vi "Plot_RT_Graph.vi"() -> ()   [LabVIEW 2017]
uses:
  <vilib>/Utility/file.llb/Read From Spreadsheet File (DBL).vi
panel:
  out "R vs T":cluster{"all rows":dbl[], "all rows":dbl[]}(graph)
  in  "stop":bool
  out "T vs t":cluster{"all rows":dbl[], "all rows":dbl[]}(graph)
  in  "file path X":path=path "c:/test.txt"
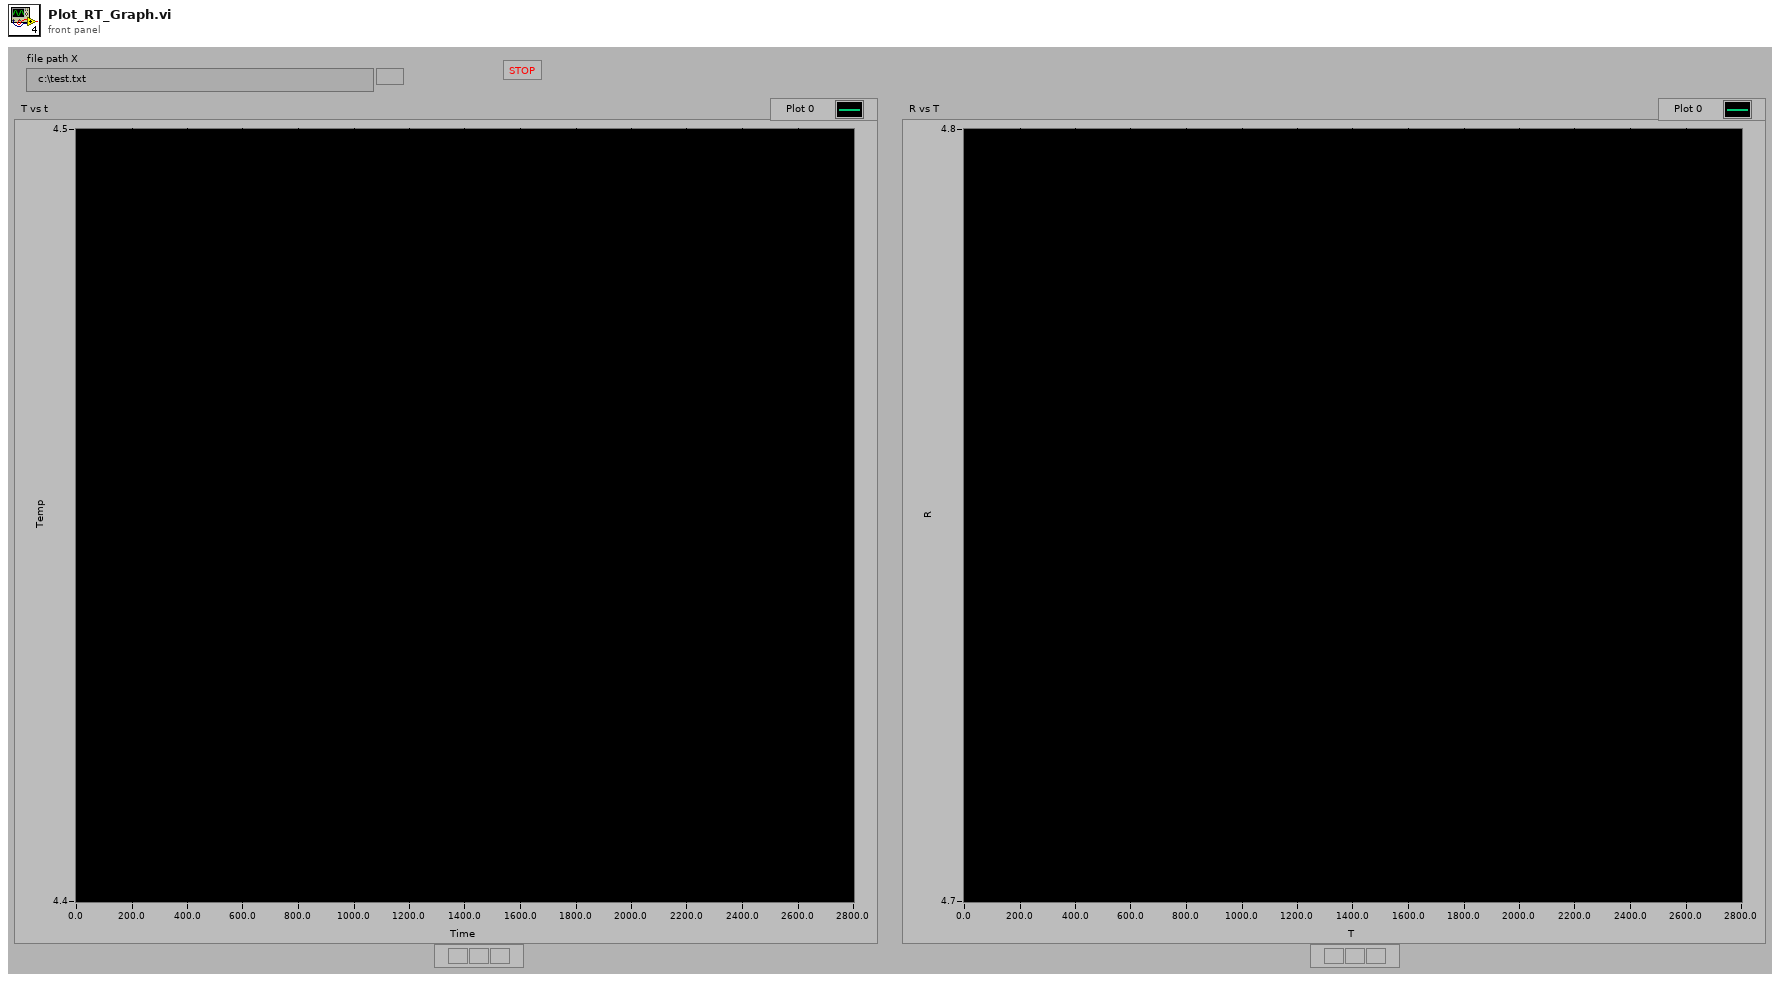
[diagram p1: front panel]
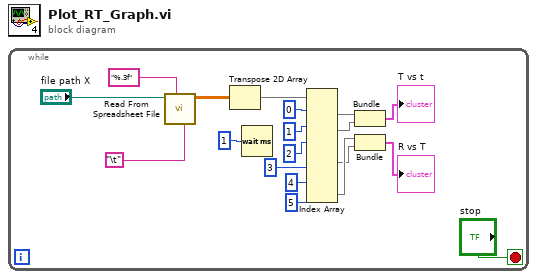
[diagram p0: block diagram]
diagram:
  n1 = while {
    stop <- "stop" stop-if-true
    n2 = call-poly <vilib>:"Read From Spreadsheet File.vi"("delimiter (\\t)"="\t" ("delimiter (\\t)"), "format (%.3f)"="%.3f", "file path (dialog if empty)"="file path X") -> ("all rows"=w12:dbl[][])  [unwired: 4 in, 4 out]
    n3 = Transpose 2D Array(2D array=w12) -> (transposed array=w11:dbl[][])
    n4 = Wait (ms)(milliseconds to wait=u32 1) -> ()  [unwired: 1 out]
    n5 = Index Array(array=w11, index (row) #1=0 ("index (row)"), index (row) #2=1 ("index (row)"), index (row) #3=2 ("index (row)"), index (row) #4=3 ("index (row)"), index (col) #5=4 ("disabled index (col)"), index (col) #6=5 ("index (col)")) -> (element #1=w6:dbl[], element #2=w14:dbl[], element #4=w1:dbl[], element #6=w2:dbl[])  [unwired: 6 in, 2 out]
    n6 = Bundle(w6, w14) -> (→"T vs t":cluster{dbl[], dbl[]})  [unwired: 1 in]
    n7 = Bundle(w2, w1) -> (→"R vs T":cluster{dbl[], dbl[]})  [unwired: 1 in]
  }
